vi "readTuplaEnDB.vi"(8 "error in":errorcluster, 11 "claseDB in":refnum<class "claseDB.lvclass">) -> (0 "error out":errorcluster, 2 "dataReadingOut":string[][](array[string]), 3 "claseDB out":refnum<class "claseDB.lvclass">)   [LabVIEW 2014, in "claseDB.lvclass"]
uses:
  claseDB.lvclass
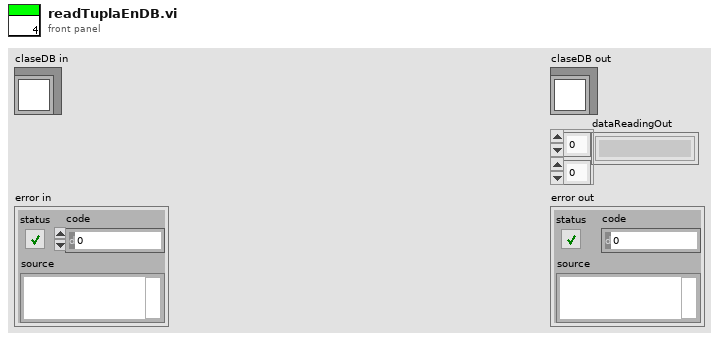
[diagram p1: front panel]
types:
  T1 = cluster{"objetoProduct":cluster{"idProduct":dbl, "od":string, "steelGrade":string, "lote":string, "dateCreate":timestamp, "idRecipe":dbl}, "objetoImage":cluster{"idImage":dbl, "camposDeMedicion":string, "dateCreate":timestamp}, "objetoRecipe":cluster{"idRecipe":dbl, "od":string, "steelGrade":string, "camposDeMedicion":string, "dateCreate":timestamp, "idStadistic":string}, "objetoStadistic":cluster{"idStadistic":dbl, "camposDeMedicion":string, "dateCreate":timestamp}, "objetoMetalRod":cluster{"idRod":dbl, "camposDeMedicion":string, "dateCreate":timestamp, "idProduct":dbl, "idImage":dbl}, "tableToUse":cluster{"useTableProduct":bool, "useTableImage":bool, "useTableRecipe":bool, "useTableStadistic":bool, "useTableMetalRod":bool}}
  T2 = cluster{"useTableProduct":bool, "useTableImage":bool, "useTableRecipe":bool, "useTableStadistic":bool, "useTableMetalRod":bool}
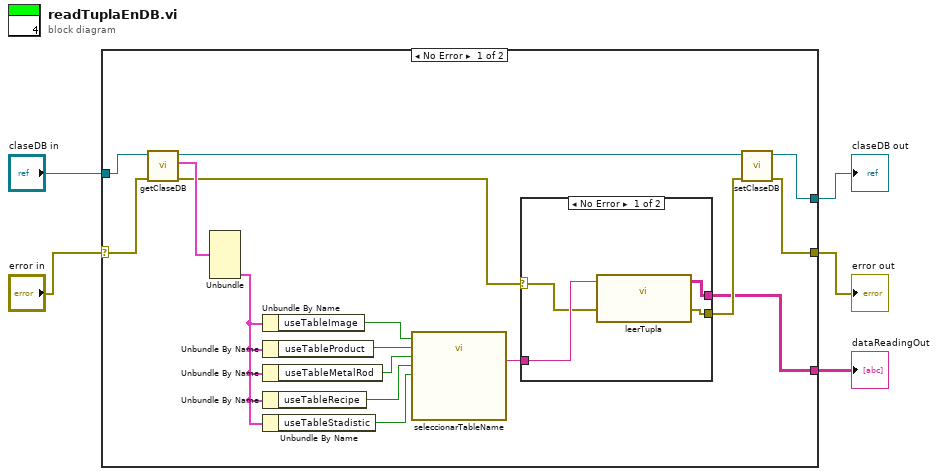
[diagram p0: block diagram]
diagram:
  n1 = case shown="No Error" "error in" {
    selector: "error in" -> [w20 w27]
    tunnel: [w18 w28] -> w4
    tunnel: "claseDB in" -> [w21 w28]
    tunnel: [w17 w27] -> w2
    tunnel: [w6 _] -> w1
    frame No Error {
      n2 = call "getClaseDB.vi"("error in"=w20, "claseDB.lvclass"=w21) -> ("error out"=w9:errorcluster, "datosClaseDB"=w16:T1, "claseDB.lvclass 2"=w19:refnum<class "claseDB.lvclass">)  [unwired: 7 in]
      n3 = Unbundle(w16) -> ("tableToUse"=w15:T2)  [unwired: 5 out]
      n4 = Unbundle By Name(w15) -> ("useTableImage"=w14:bool)
      n5 = Unbundle By Name(w15) -> ("useTableProduct"=w13:bool)
      n6 = Unbundle By Name(w15) -> ("useTableMetalRod"=w12:bool)
      n7 = Unbundle By Name(w15) -> ("useTableRecipe"=w11:bool)
      n8 = Unbundle By Name(w15) -> ("useTableStadistic"=w10:bool)
      n9 = call "seleccionarTableName.vi"("stadisticTable?"=w10, "recipeTable?"=w11, "metalrodTable?"=w12, "productTable?"=w13, "imageTable?"=w14) -> ("tableNameOut"=w8:string)  [unwired: 6 in]
      n10 = case shown="No Error" w9 {
        selector: w9 -> [w24 w26]
        tunnel: w8 -> [w25 _]
        tunnel: [w23 w26] -> w7
        tunnel: [w22 _] -> w6
        frame No Error {
          n11 = call "leerTupla.vi"("error in"=w24, "tableName"=w25) -> ("error out"=w23:errorcluster, "dataReadingOut"=w22:string[][])  [unwired: 7 in, 1 out]
        }
        frame Error {
        }
      }
      n12 = call "setClaseDB.vi"("error in"=w7, "claseDB in"=w19) -> ("error out"=w17:errorcluster, "claseDB out"=w18:refnum<class "claseDB.lvclass">)  [unwired: 8 in]
    }
    frame Error {
    }
  }
  "claseDB out" <- w4
  "error out" <- w2
  "dataReadingOut" <- w1
